vi "_PM[RADICAL]_.vi"() -> ()   [LabVIEW 2011]
uses:
  <vilib>/Utility/file.llb/Write To Spreadsheet File (DBL).vi
panel:
  out "数値 2":dbl format="%#_4g"
  in  "HOT/COLD":bool
  in  "Control":T1={"GPIB_ATT"="28", "6501Dev#"=1, "GPIB_SP"="18", "GPIB_PM"="13", "GPIB_DSA"="11", "GPIB_DMM (TPD)"="23", "GPIB_MPI"="2", "mortor設定"=[{"Axis"=0, "ID"=0, "HIspeed"=200.0, "LOspeed"=100.0, "ACCEL(ms)"=100.0, "Sratio"=50.0, "フリーラン\n"=FALSE, "文字列"="DSB HOT/COLD"}, {"Axis"=1, "ID"=0, "HIspeed"=4.0, "LOspeed"=4.0, "ACCEL(ms)"=100.0, "Sratio"=50.0, "フリーラン\n"=TRUE, "文字列"="SubMM Att"}, {"Axis"=0, "ID"=0, "HIspeed"=200.0, "LOspeed"=100.0, "ACCEL(ms)"=100.0, "Sratio"=50.0, "フリーラン\n"=TRUE, "文字列"="MPI Port1"}, {"Axis"=1, "ID"=0, "HIspeed"=200.0, "LOspeed"=100.0, "ACCEL(ms)"=100.0, "Sratio"=50.0, "フリーラン\n"=TRUE, "文字列"="MPI Port2"}, {"Axis"=1, "ID"=0, "HIspeed"=200.0, "LOspeed"=100.0, "ACCEL(ms)"=100.0, "Sratio"=50.0, "フリーラン\n"=TRUE, "文字列"="gainComp"}], "DATAパス"=path "C:/Documents and Settings/鵜澤佳徳/デスクトップ/data/プロトカートリッジ/110113_protoC4-9/110127_mixtest", "DBパス "=path "Z:/band10/Labview_ALMA/MIX95/test", "comment"="mix10test", "ColdCarts"="003601", "Th"=300.0, "Tc"=77.0, "Set_SIS_volt"=2.0999999046325684, "Offset"=0.0, "control"=0, "FreqLO"=874.0, "Set_Mag_Cur"=800.0, "MPI offset(mm)"=22.962, "HOT/COLD"=0} {"HOT/COLD" items=["DSB", "SBR (Cart.)", "GainComp", "SBR (MIX)"]; "control" items=["CLOSE LOOP", "OPEN LOOP", "Not Control"]}
  in  "数値":i32=300
  out "波形チャート":dbl(graph)
  in  "停止":bool
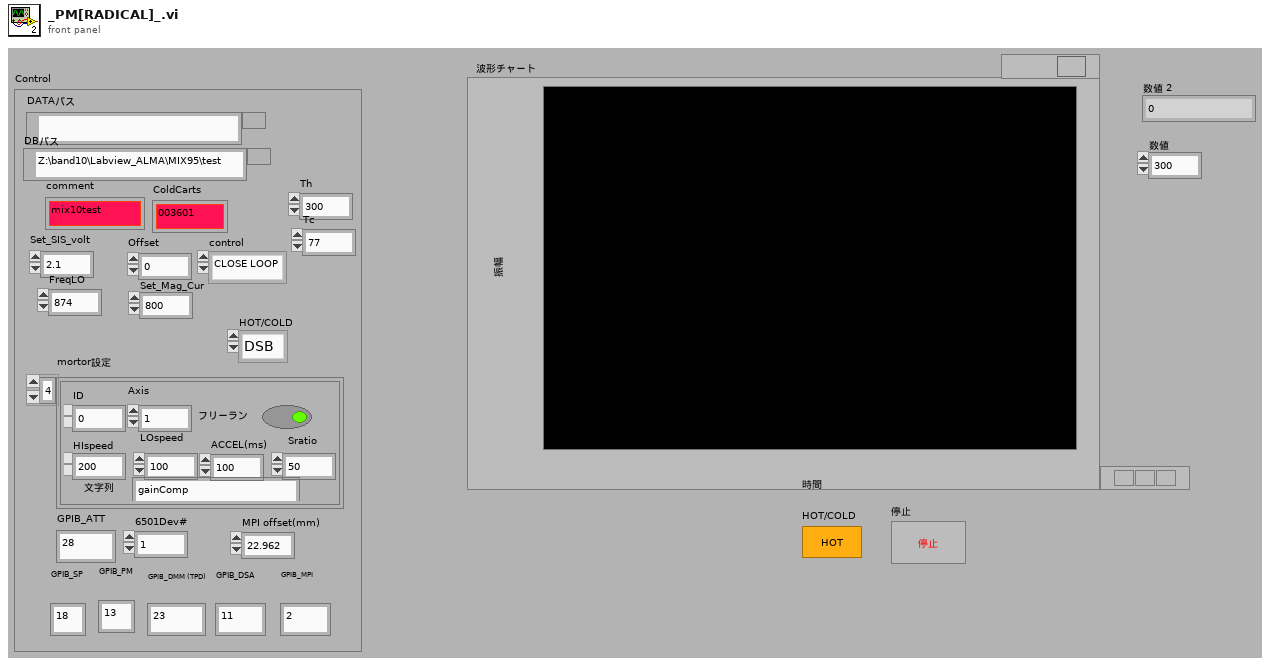
[diagram p1: front panel]
types:
  T1 = cluster{"GPIB_ATT":string, "6501Dev#":i16, "GPIB_SP":string, "GPIB_PM":string, "GPIB_DSA":string, "GPIB_DMM (TPD)":string, "GPIB_MPI":string, "mortor設定":cluster{"Axis":i16, "ID":i16, "HIspeed":dbl, "LOspeed":dbl, "ACCEL(ms)":dbl, "Sratio":dbl, "フリーラン\n":bool, "文字列":string}[], "DATAパス":path, "DBパス ":path, "comment":string, "ColdCarts":string, "Th":dbl, "Tc":dbl, "Set_SIS_volt":dbl, "Offset":dbl, "control":u16, "FreqLO":dbl, "Set_Mag_Cur":dbl, "MPI offset(mm)":dbl, "HOT/COLD":u16}
  T2 = cluster{"Axis":i16, "ID":i16, "HIspeed":dbl, "LOspeed":dbl, "ACCEL(ms)":dbl, "Sratio":dbl, "フリーラン\n":bool, "文字列":string}[]
  T3 = cluster{"Axis":i16, "ID":i16, "HIspeed":dbl, "LOspeed":dbl, "ACCEL(ms)":dbl, "Sratio":dbl, "フリーラン\n":bool, "文字列":string}
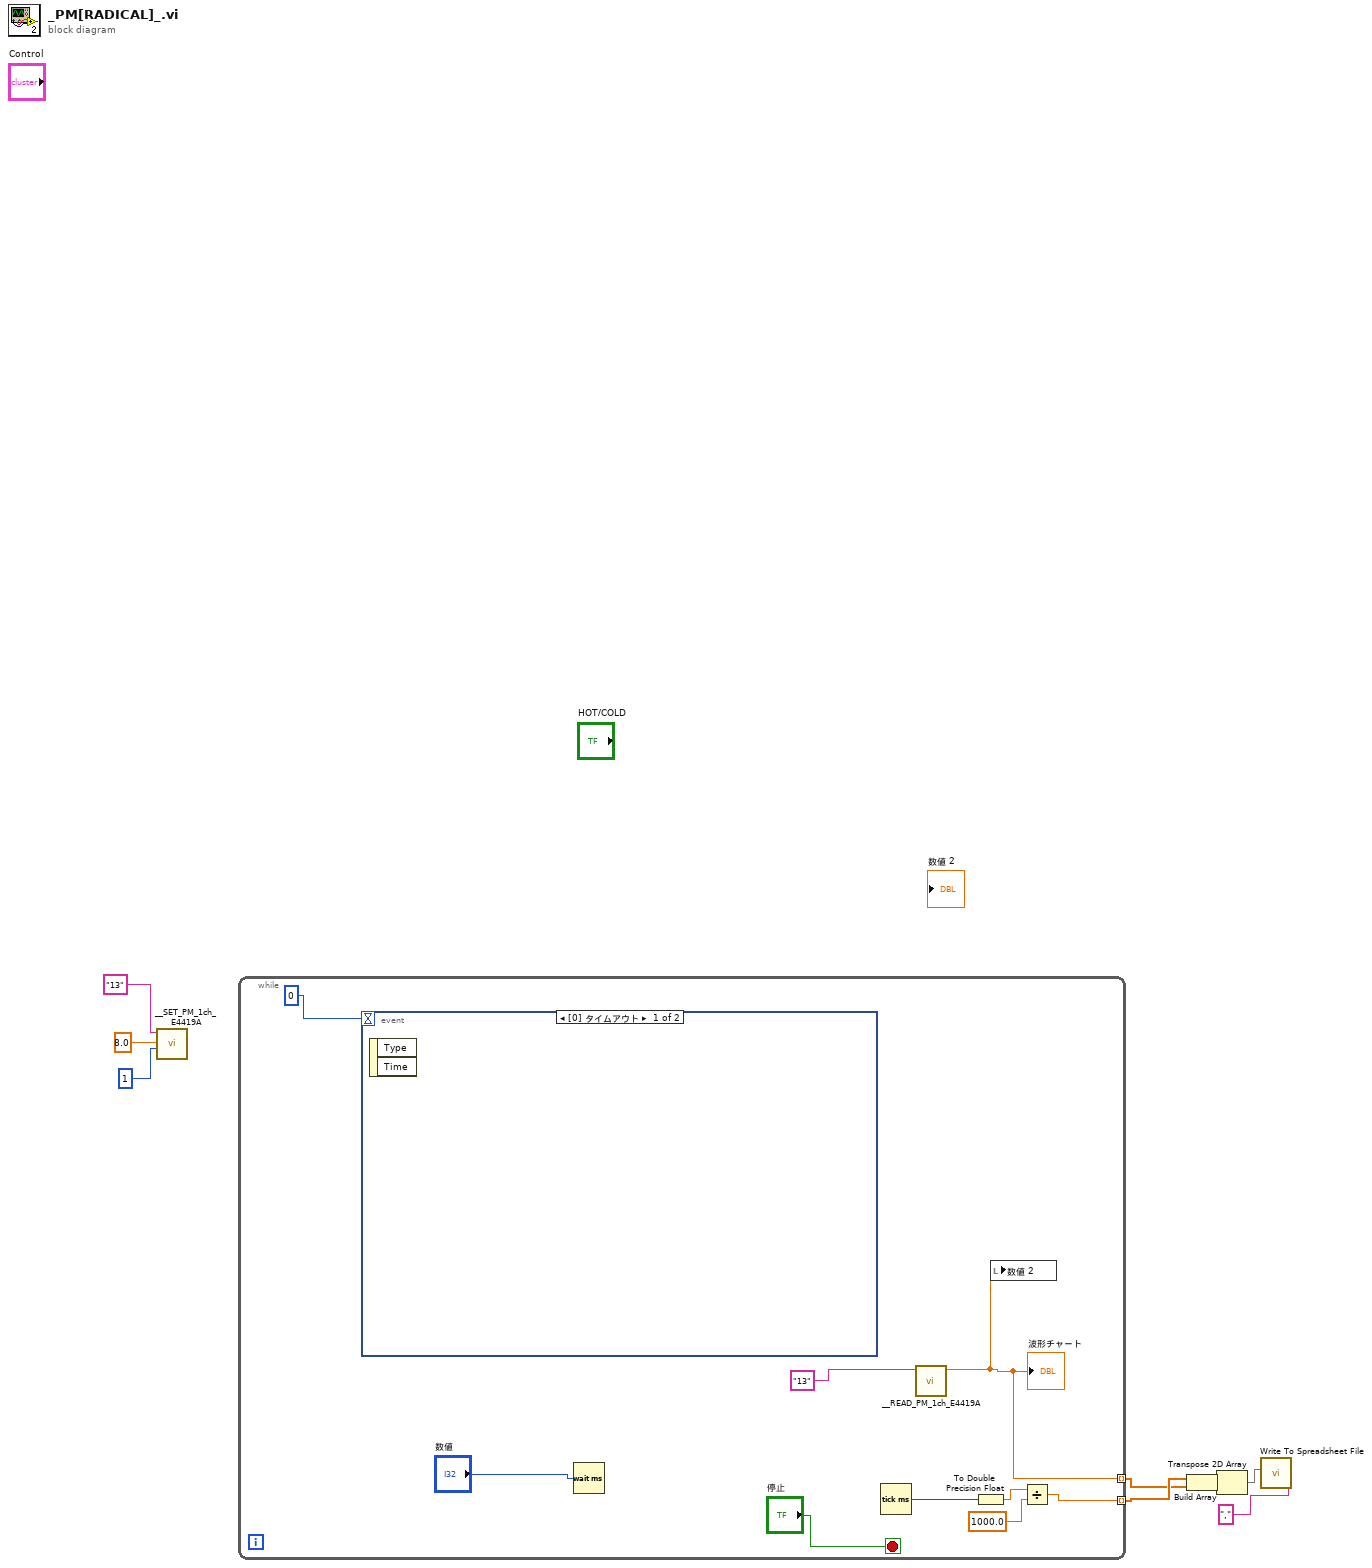
[diagram p0: block diagram]
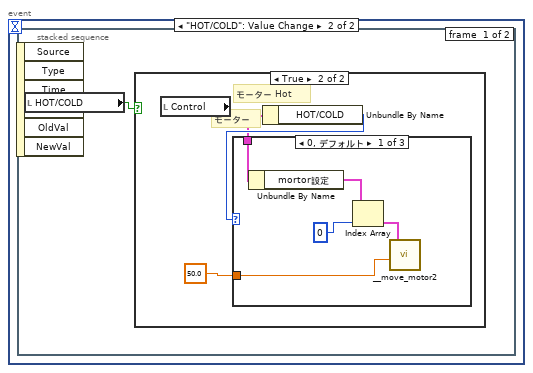
[diagram p2: hidden frame]
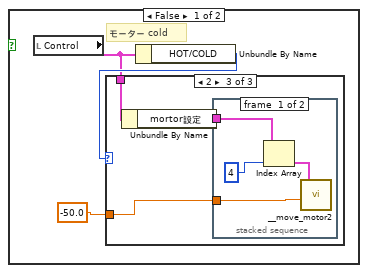
[diagram p3: hidden frame]
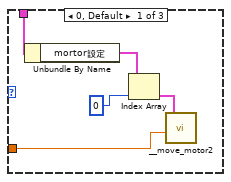
[diagram p4: hidden frame]
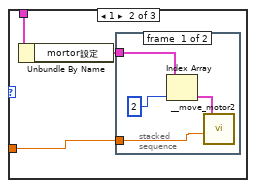
[diagram p5: hidden frame]
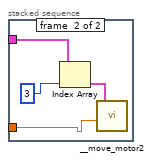
[diagram p6: hidden frame]
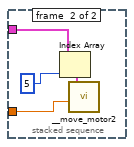
[diagram p7: hidden frame]
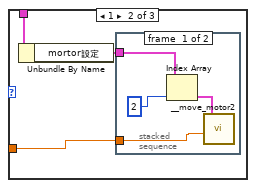
[diagram p8: hidden frame]
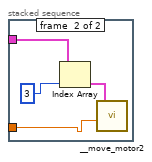
[diagram p9: hidden frame]
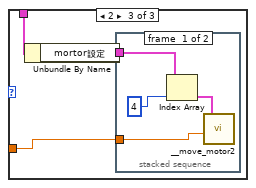
[diagram p10: hidden frame]
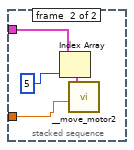
[diagram p11: hidden frame]
diagram:
  n1 = call "__SET_PM_1ch_E4419A.VI"("aveg"=1, "frq(GHz)"=8.0, "GPIB"="13") -> ()  [unwired: 5 in]
  n2 = while {
    tunnel: [w9] -> w1 mode=indexing
    tunnel: [w12] -> w2 mode=indexing
    stop <- "停止" stop-if-true
    n3 = event shown="[0] タイムアウト" {
      selector: _ -> [_ _]
      dyn-events: _ -> [_ _]
      timeout: 0 -> [_ _]
      event Timeout {
        n4 = event-data() -> ()  [unwired: 1 in, 2 out]
      }
      event "HOT/COLD": Value Change {
        n5 = event-data() -> ()  [unwired: 1 in, 6 out]
        n6 = stacked-sequence {
          frame #0 {
            n7 = local read "HOT/COLD"() -> (w18:bool)
            n8 = case shown="TRUE" w18 {
              frame False {
                # "モーター cold"
                n9 = local read "Control"() -> (w19:T1)
                n10 = Unbundle By Name(w19) -> ("HOT/COLD"=w20:u16)
                n11 = case shown="2" w20 {
                  tunnel: w19 -> [w25 w29 w40]
                  tunnel: -50.0 -> [w22 w27 w38]
                  frame 0, Default {
                    n12 = Unbundle By Name(w25) -> ("mortor設定"=w24:T2)
                    n13 = Index Array(array=w24, index=0) -> (element=w23:T3)
                    n14 = call "__move_motor2.vi"("移動距離"=w22, "motor設定"=w23) -> ()  [unwired: 2 in, 2 out]
                  }
                  frame 1 {
                    n15 = Unbundle By Name(w29) -> ("mortor設定"=w28:T2)
                    n16 = stacked-sequence {
                      tunnel: w28 -> [w32 w36]
                      tunnel: w27 -> [w30 w34]
                      frame #0 {
                        n17 = Index Array(array=w32, index=2) -> (element=w31:T3)
                        n18 = call "__move_motor2.vi"("移動距離"=w30, "motor設定"=w31) -> ()  [unwired: 2 in, 2 out]
                      }
                      frame #1 {
                        n19 = Index Array(array=w36, index=3) -> (element=w35:T3)
                        n20 = call "__move_motor2.vi"("移動距離"=w34, "motor設定"=w35) -> ()  [unwired: 2 in, 2 out]
                      }
                    }
                  }
                  frame 2 {
                    n21 = Unbundle By Name(w40) -> ("mortor設定"=w39:T2)
                    n22 = stacked-sequence {
                      tunnel: w39 -> [w43 w47]
                      tunnel: w38 -> [w41 w45]
                      frame #0 {
                        n23 = Index Array(array=w43, index=4) -> (element=w42:T3)
                        n24 = call "__move_motor2.vi"("移動距離"=w41, "motor設定"=w42) -> ()  [unwired: 2 in, 2 out]
                      }
                      frame #1 {
                        n25 = Index Array(array=w47, index=5) -> (element=w46:T3)
                        n26 = call "__move_motor2.vi"("移動距離"=w45, "motor設定"=w46) -> ()  [unwired: 2 in, 2 out]
                      }
                    }
                  }
                }
              }
              frame True {
                # "モーター Hot"
                # "モーター"
                n27 = local read "Control"() -> (w49:T1)
                n28 = Unbundle By Name(w49) -> ("HOT/COLD"=w50:u16)
                n29 = case shown="0, デフォルト" w50 {
                  tunnel: w49 -> [w55 w59 w70]
                  tunnel: 50.0 -> [w52 w57 w68]
                  frame 0, Default {
                    n30 = Unbundle By Name(w55) -> ("mortor設定"=w54:T2)
                    n31 = Index Array(array=w54, index=0) -> (element=w53:T3)
                    n32 = call "__move_motor2.vi"("移動距離"=w52, "motor設定"=w53) -> ()  [unwired: 2 in, 2 out]
                  }
                  frame 1 {
                    n33 = Unbundle By Name(w59) -> ("mortor設定"=w58:T2)
                    n34 = stacked-sequence {
                      tunnel: w58 -> [w62 w66]
                      tunnel: w57 -> [w60 w64]
                      frame #0 {
                        n35 = Index Array(array=w62, index=2) -> (element=w61:T3)
                        n36 = call "__move_motor2.vi"("移動距離"=w60, "motor設定"=w61) -> ()  [unwired: 2 in, 2 out]
                      }
                      frame #1 {
                        n37 = Index Array(array=w66, index=3) -> (element=w65:T3)
                        n38 = call "__move_motor2.vi"("移動距離"=w64, "motor設定"=w65) -> ()  [unwired: 2 in, 2 out]
                      }
                    }
                  }
                  frame 2 {
                    n39 = Unbundle By Name(w70) -> ("mortor設定"=w69:T2)
                    n40 = stacked-sequence {
                      tunnel: w69 -> [w73 w77]
                      tunnel: w68 -> [w71 w75]
                      frame #0 {
                        n41 = Index Array(array=w73, index=4) -> (element=w72:T3)
                        n42 = call "__move_motor2.vi"("移動距離"=w71, "motor設定"=w72) -> ()  [unwired: 2 in, 2 out]
                      }
                      frame #1 {
                        n43 = Index Array(array=w77, index=5) -> (element=w76:T3)
                        n44 = call "__move_motor2.vi"("移動距離"=w75, "motor設定"=w76) -> ()  [unwired: 2 in, 2 out]
                      }
                    }
                  }
                }
              }
            }
          }
          frame #1 {
          }
        }
      }
    }
    n45 = Wait (ms)(milliseconds to wait="数値") -> ()  [unwired: 1 out]
    n46 = Tick Count (ms)() -> (millisecond timer value=w13:u32)
    n47 = call "__READ_PM_1ch_E4419A.VI"("GPIB"="13") -> ("chA"=w9:dbl)  [unwired: 6 in]
    "波形チャート" <- w9
    n48 = To Double Precision Float(number=w13) -> (double precision float=w11:dbl)
    n49 = local write "数値 2"(w9) -> ()
    n50 = Divide(x=w11, y=1000.0) -> (x/y=w12:dbl)
  }
  n51 = Build Array(w2, w1) -> (w5:dbl[][])
  n52 = Transpose 2D Array(2D array=w5) -> (transposed array=w3:dbl[][])
  n53 = call-poly <vilib>:"Write To Spreadsheet File.vi"("delimiter (\\t)"=",", "2D data"=w3) -> ()  [unwired: 6 in, 1 out]
